vi "arduinoInitGlobalVariables.vi"() -> ()   [LabVIEW 2012]
uses:
  GlobalLB.vi
panel:
  in  "LB status":bool[](array[boolean])=[FALSE, FALSE, FALSE, FALSE]
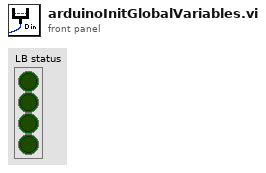
[diagram p1: front panel]
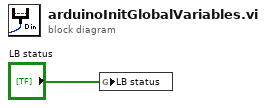
[diagram p0: block diagram]
diagram:
  n1 = global write "GlobalLB.vi" "LB status"("LB status") -> ()
